vi "Reactor Temperature Rise Redundancy.vi"(0 "SI100_ReactorTemperatureRise.lvclass":refnum<class "ReactorTemperatureRise.lvclass">, 1 "3 JEC CT951 XQ01":dbl, 2 "3 JEC CT952 XQ01":dbl, 3 "3 JEC CT953 XQ01":dbl, 4 "3 JEC CT954 XQ01":dbl, 5 "error in":errorcluster, 8 "Redundancy":enum16{"R1", "R2", "R3", "R4"}(ring)) -> (14 "SI100_ReactorTemperatureRise.lvclass 2":refnum<class "ReactorTemperatureRise.lvclass">, 15 "Avg Temp Rise":dbl, 16 "T-Rise 2nd Max":dbl, 19 "error IO":errorcluster)   [LabVIEW 2022 SP3, in "ReactorTemperatureRise.lvclass"]
uses:
  ReactorTemperatureRise.lvclass
  ReactorTemperatureRise.lvclass/ReactorTemperatureRise.ctl
panel:
  # "SI100"
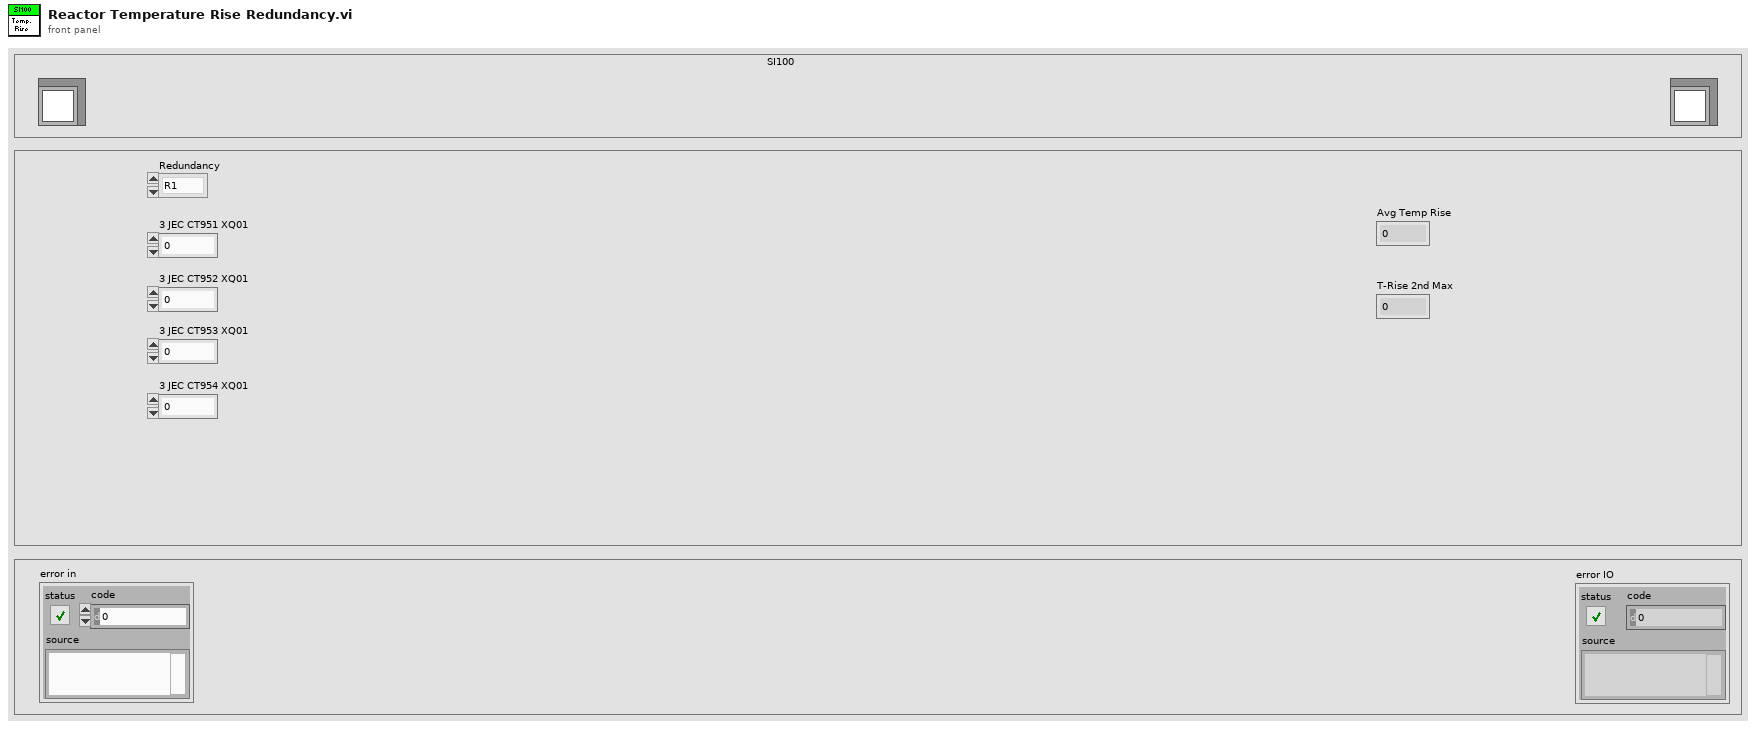
[diagram p1: front panel]
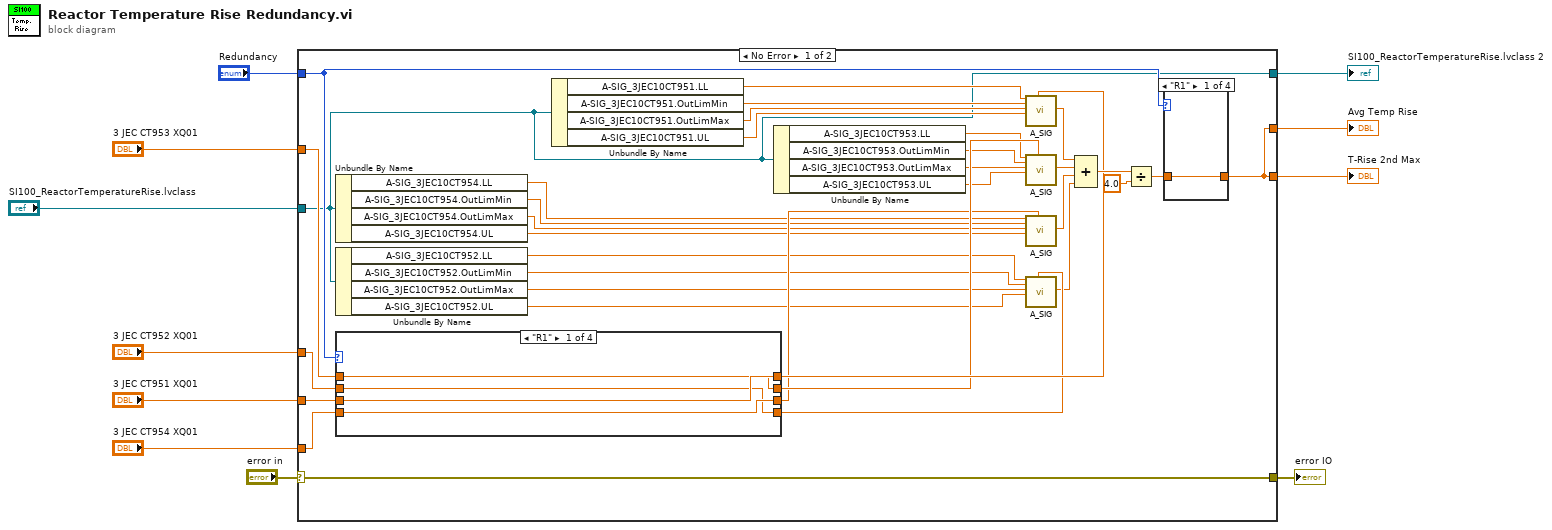
[diagram p0: block diagram]
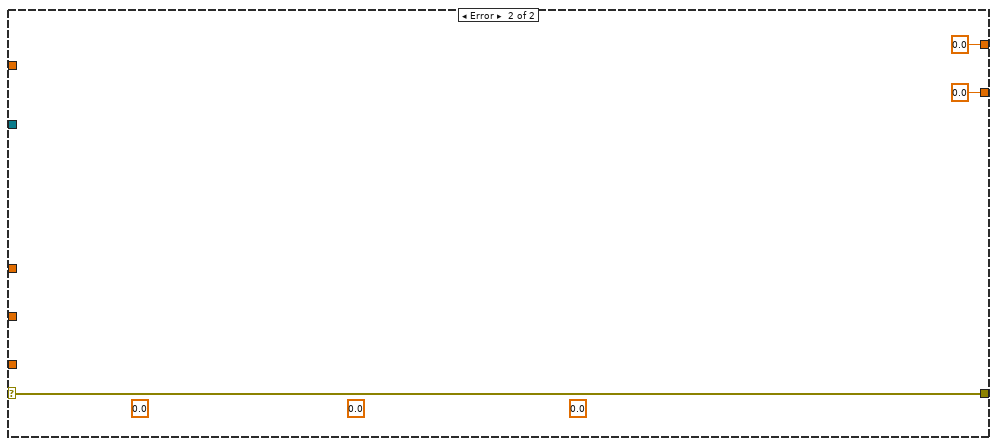
[diagram p8: hidden frame]
diagram:
  n1 = case shown="No Error" "error in" {
    selector: "error in" -> [w44 w67]
    tunnel: [w12 0.0] -> w11
    tunnel: [w12 0.0 ("AP2")] -> w9
    tunnel: [w44 w67] -> w8
    tunnel: "SI100_ReactorTemperatureRise.lvclass" -> [w14 _]
    tunnel: [w14 _] -> w6
    tunnel: "Redundancy" -> [w31 _]
    tunnel: "3 JEC CT951 XQ01" -> [w43 _]
    tunnel: "3 JEC CT952 XQ01" -> [w42 _]
    tunnel: "3 JEC CT953 XQ01" -> [w41 _]
    tunnel: "3 JEC CT954 XQ01" -> [w40 _]
    frame No Error {
      n2 = Unbundle By Name(w14) -> ("A-SIG_3JEC10CT954.LL"=w22:dbl, "A-SIG_3JEC10CT954.OutLimMin"=w21:dbl, "A-SIG_3JEC10CT954.OutLimMax"=w20:dbl, "A-SIG_3JEC10CT954.UL"=w19:dbl)
      n3 = Unbundle By Name(w14) -> ("A-SIG_3JEC10CT952.LL"=w18:dbl, "A-SIG_3JEC10CT952.OutLimMin"=w17:dbl, "A-SIG_3JEC10CT952.OutLimMax"=w16:dbl, "A-SIG_3JEC10CT952.UL"=w15:dbl)
      n4 = case shown="\"R1\"" w31 {
        tunnel: w43 -> [w54 w57 w60 w63]
        tunnel: w42 -> [w51 w58 w61 w64]
        tunnel: w41 -> [w53 w56 w59 w66]
        tunnel: w40 -> [w52 w55 w62 w65]
        tunnel: [w54 w58 w62 w66] -> w39
        tunnel: [w53 w57 w61 w65] -> w38
        tunnel: [w52 w56 w60 w64] -> w37
        tunnel: [w51 w55 w59 w63] -> w36
        frame "R1" {
        }
        frame "R2" {
        }
        frame "R3" {
        }
        frame "R4" {
        }
      }
      n5 = Unbundle By Name(w14) -> ("A-SIG_3JEC10CT951.LL"=w30:dbl, "A-SIG_3JEC10CT951.OutLimMin"=w29:dbl, "A-SIG_3JEC10CT951.OutLimMax"=w28:dbl, "A-SIG_3JEC10CT951.UL"=w27:dbl)
      n6 = Unbundle By Name(w14) -> ("A-SIG_3JEC10CT953.LL"=w26:dbl, "A-SIG_3JEC10CT953.OutLimMin"=w25:dbl, "A-SIG_3JEC10CT953.OutLimMax"=w24:dbl, "A-SIG_3JEC10CT953.UL"=w23:dbl)
      n7 = call "A_SIG.vi"("LL"=w30, "OutLimMin"=w29, "OutLimMax"=w28, "UL"=w27, "Input"=w39) -> ("A_SIG_out"=w35:dbl)  [unwired: 13 in, 1 out]
      n8 = call "A_SIG.vi"("LL"=w26, "OutLimMin"=w25, "OutLimMax"=w24, "UL"=w23, "Input"=w38) -> ("A_SIG_out"=w34:dbl)  [unwired: 13 in, 1 out]
      n9 = call "A_SIG.vi"("LL"=w22, "OutLimMin"=w21, "OutLimMax"=w20, "UL"=w19, "Input"=w37) -> ("A_SIG_out"=w33:dbl)  [unwired: 13 in, 1 out]
      n10 = call "A_SIG.vi"("LL"=w18, "OutLimMin"=w17, "OutLimMax"=w16, "UL"=w15, "Input"=w36) -> ("A_SIG_out"=w32:dbl)  [unwired: 13 in, 1 out]
      n11 = Compound Arithmetic op=ADD(w35, w34, w33, w32) -> (w46:dbl)
      n12 = Divide(x=w46, y=4.0) -> (x/y=w13:dbl)
      n13 = case shown="\"R1\"" w31 {
        tunnel: w13 -> [w47 w48 w49 w50]
        tunnel: [w47 w48 w49 w50] -> w12
        frame "R1" {
        }
        frame "R2" {
        }
        frame "R3" {
        }
        frame "R4" {
        }
      }
    }
    frame Error {
      (unwired) 0.0 ("AP2")
      (unwired) 0.0 ("AP2")
      (unwired) 0.0 ("AP1")
    }
  }
  "T-Rise 2nd Max" <- w11
  "Avg Temp Rise" <- w9
  "error IO" <- w8
  "SI100_ReactorTemperatureRise.lvclass 2" <- w6
